vi "Loop_SM.vi"() -> ()   [LabVIEW 2017, in "WCDrive2018.lvlib"]
uses:
  WCDrive2018.lvlib
  ProtoType Code/EXAMPLE 2017 competition code/roboRIO Code/TypeDefs/Cluster_PID Constants Standard.ctl
  Cluster_Auto Shut Off Ranges.ctl
  ENUM_State.ctl
  Enum_SM Cmd Select.ctl
  ENUM_Action.ctl
  Enum Tab_Select PID Mode.ctl
  Cluster_SM to HW Data.ctl
  Enum_HW Cmd Select.ctl
  Cluster_CMD to SM Data.ctl
  Cluster_HW Status.ctl
  ProtoType Code/EXAMPLE 2017 competition code/roboRIO Code/TypeDefs/Cluster_SRX Status With Encoder.ctl
  Cluster_SM Status.ctl
  <vilib>/Rock Robotics/WPI/ThirdParty/Sensors/navX/_TypeDefs/FRIC_navX_DeviceNumbersTypeDef.ctl
  Global_CMD to SM Data.vi
  Global_HW_Status Out.vi
  _SHARE ALL/Global Share All/Global_STOP.vi
  <vilib>/addons/control/pid/pid.llb/PID (DBL).vi
  Global_SM Out Data.vi
  <vilib>/addons/control/pid/NI_PID_pid.lvlib
panel:
  out "Drive_HW_Status":T1
  out "SM Cmd":T3
  out "HW Cmd Out":T5
  in  "PID Select":T7
  in  "PID Track Rotation":T8={"proportional gain (Kc)"=0.005, "integral time (Ti, min)"=0.0, "derivative time (Td, min)"=0.0028} {"derivative time (Td, min)" format="%.5f"; "integral time (Ti, min)" format="%.5f"; "proportional gain (Kc)" format="%.5f"}
  in  "PID Lock Angle Rotation":T8={"proportional gain (Kc)"=0.012, "integral time (Ti, min)"=0.0, "derivative time (Td, min)"=0.002} {"derivative time (Td, min)" format="%.5f"; "integral time (Ti, min)" format="%.5f"; "proportional gain (Kc)" format="%.5f"}
  in  "PID Track Distance":T8={"proportional gain (Kc)"=0.005, "integral time (Ti, min)"=0.0, "derivative time (Td, min)"=0.0} {"derivative time (Td, min)" format="%.5f"; "integral time (Ti, min)" format="%.5f"; "proportional gain (Kc)" format="%.5f"}
  out "Action":T9
  out "CMDMODE":T4
  out "Complete":bool
  out "PID Output":dbl
  out "PID Reading":dbl
  out "PID Target":dbl
  out "Cycle Time":dbl
  out "State":T10
  out "Output":dbl(graph)
  out "Process Chart":cluster{"PID Target":dbl, "PID Reading":dbl}(graph)
  in  "Auto Shut Off Ranges":T11={"Track Front Back"=1.0, "Track Rotation"=1.0, "Track Lateral"=1.0, "Track Vision"=2.0}
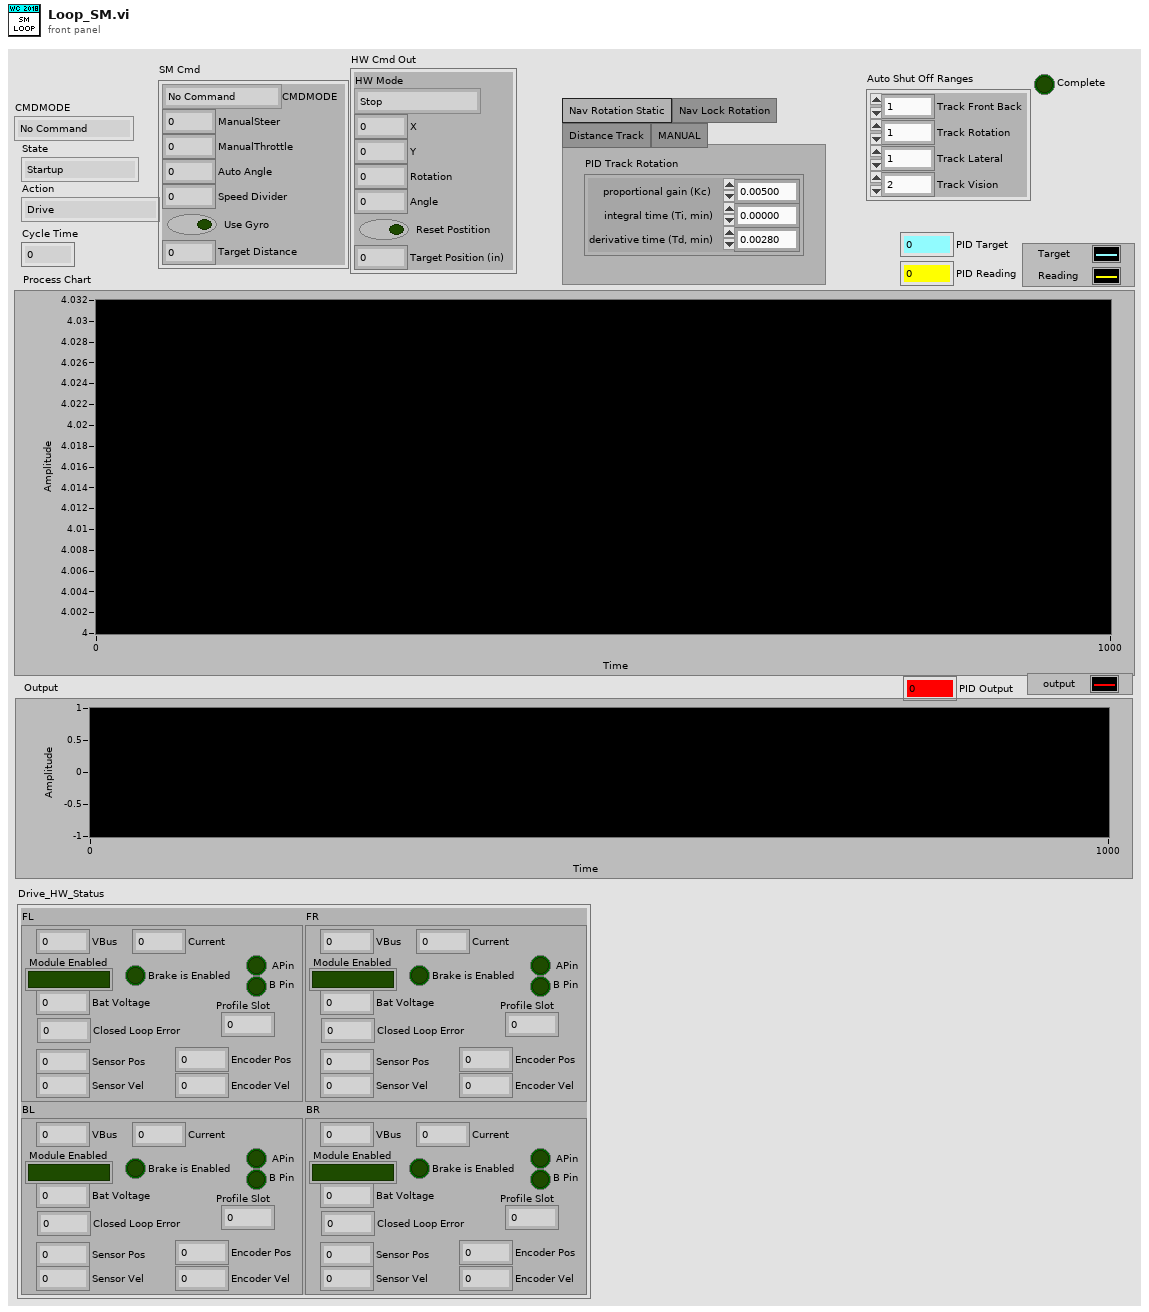
[diagram p1: front panel]
types:
  T1 = typedef "WCDrive2018.lvlib/Cluster_HW Status.ctl" = cluster{"BL":T2, "BR":T2, "FL":T2, "FR":T2}
  T2 = typedef "Cluster_SRX Status With Encoder.ctl" = cluster{"VBus ":dbl, "Module Enabled":bool, "Closed Loop Error":dbl, "Sensor Pos":dbl, "Sensor Vel":dbl, "Current":dbl, "Brake is Enabled":bool, "Encoder Pos":dbl, "Encoder Vel":dbl, " APin":bool, "B Pin":bool, "Bat Voltage":dbl, "Profile Slot":dbl}
  T3 = typedef "WCDrive2018.lvlib/Cluster_CMD to SM Data.ctl" = cluster{"CMDMODE":T4, "ManualSteer":dbl, "ManualThrottle":dbl, "Auto Angle":dbl, "Speed Divider":dbl, "Use Gyro":bool, "Target Distance":dbl}
  T4 = typedef "WCDrive2018.lvlib/Enum_SM Cmd Select.ctl" = enum16{"No Command", "Halt", "Manual Keep Rotation", "Manual", "Track Front", "Track Rotation"}
  T5 = typedef "WCDrive2018.lvlib/Cluster_SM to HW Data.ctl" = cluster{"HW Mode":T6, "X":dbl, "Y":dbl, "Rotation":dbl, "Angle":dbl, "Reset Postition":bool, "Target Position (in)":dbl}
  T6 = typedef "WCDrive2018.lvlib/Enum_HW Cmd Select.ctl" = enum16{"Stop", "Vbus", "Positon Lateral", "Postition  FrontBack"}
  T7 = typedef "WCDrive2018.lvlib/Enum Tab_Select PID Mode.ctl" = enum32{"Nav Rotation Static", "Nav Lock Rotation", "Distance Track", "MANUAL"}
  T8 = typedef "Cluster_PID Constants Standard.ctl" = cluster{"proportional gain (Kc)":dbl, "integral time (Ti, min)":dbl, "derivative time (Td, min)":dbl}
  T9 = typedef "WCDrive2018.lvlib/ENUM_Action.ctl" = enum16{"Drive", "No Action", "Manuel Keep Rotation", "Reset Time", "Stop Move", "Track Front Distance", "Set Lock Angle", "Reset Gyro", "Track Rotation", "NavX Pos Reset", "Reset Position"}
  T10 = typedef "WCDrive2018.lvlib/ENUM_State.ctl" = enum16{"Startup", "Idle", "Manual", "Rotation Tracking", "Distance Tracking", "Shutdown", "Manual Keep Rotation", "Halt"}
  T11 = typedef "WCDrive2018.lvlib/Cluster_Auto Shut Off Ranges.ctl" = cluster{"Track Front Back":dbl, "Track Rotation":dbl, "Track Lateral":dbl, "Track Vision":dbl}
  T12 = typedef "WCDrive2018.lvlib/Cluster_SM Status.ctl" = cluster{"Drive Cmd":T4, "Complete":bool}
  T13 = cluster{"Velocity X":dbl, "Velocity Y":dbl, "Velocity Z":dbl, "Displacement X":dbl, "Displacement Y":dbl, "Displacement Z":dbl}
  T14 = cluster{"Actions":T9[], "State":T10, "Current Time":timestamp, "Start Time":timestamp, "Loop Time (ms)":u32, "CMD Drive":T3, "Set Angle Out":dbl, "Sonar Distance":dbl, "Lock Angle":dbl, "previous State":T10, "Position Data":cluster{"Velocity X":dbl, "Velocity Y":dbl, "Velocity Z":dbl, "Displacement X":dbl, "Displacement Y":dbl, "Displacement Z":dbl}, "Shut Off Ranges":T11, "Status OUT":T12, "PID Target":dbl, "PID Reading":dbl, "PID Output":dbl, "DriveHWCmd":T5, "Gyro Angle":dbl, "Drive HW Status":T1, "PID Select":T7}
  T15 = typedef "FRIC_navX_DeviceNumbersTypeDef.ctl" = enum16{"Dev0", "Dev1", "Dev2", "Dev3"}
  T16 = cluster{"Yaw":dbl, "Roll":dbl, "Pitch":dbl, "Heading":dbl, "Fused Heading":dbl}
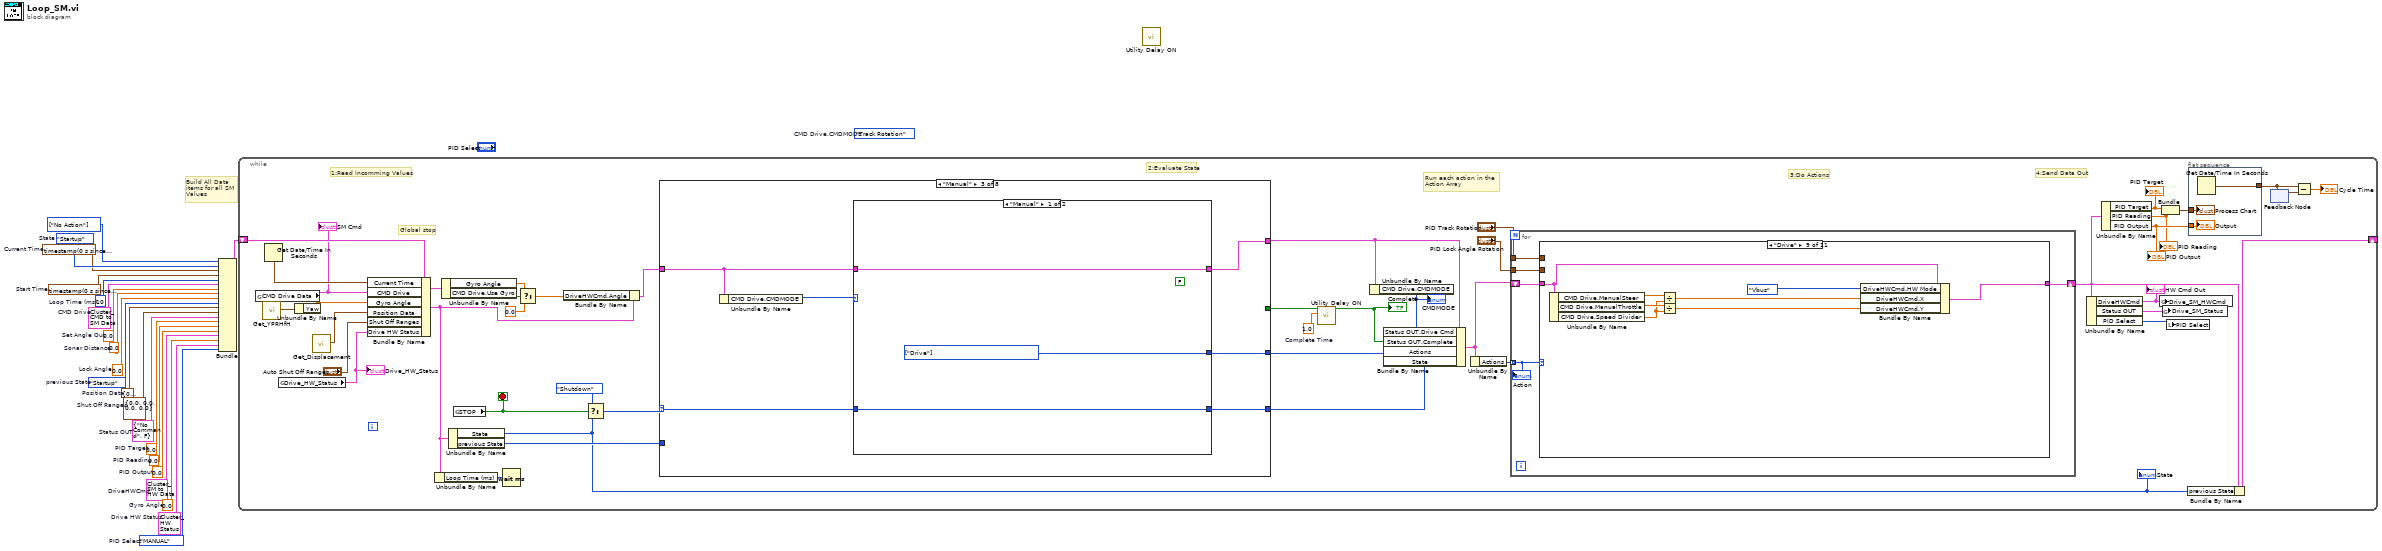
[diagram p0: block diagram]
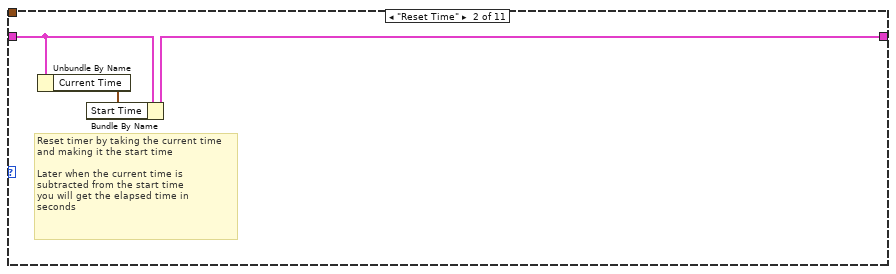
[diagram p3: hidden frame]
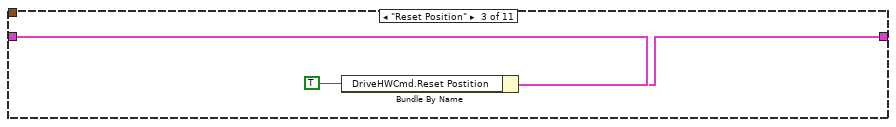
[diagram p4: hidden frame]
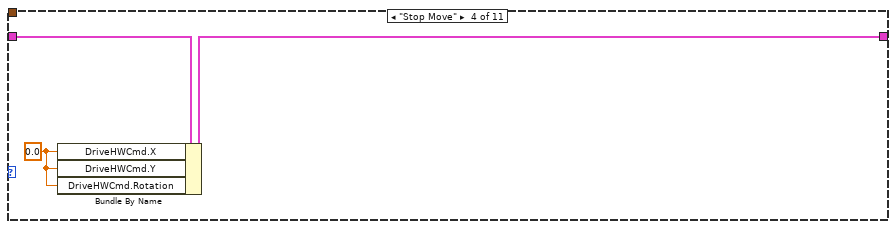
[diagram p5: hidden frame]
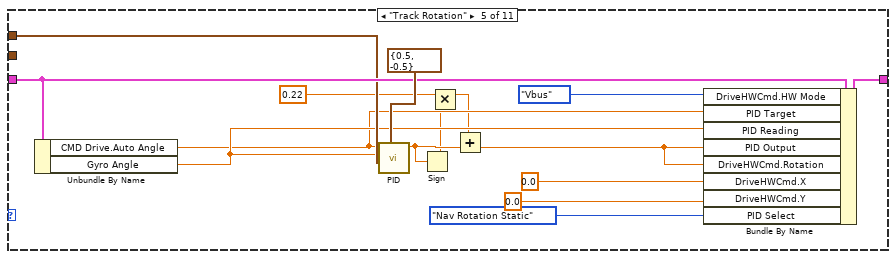
[diagram p6: hidden frame]
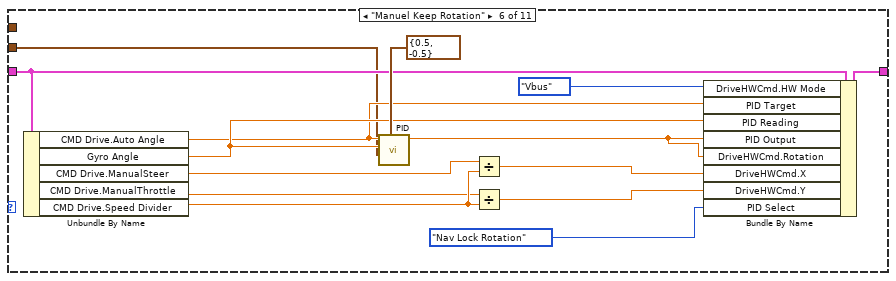
[diagram p7: hidden frame]
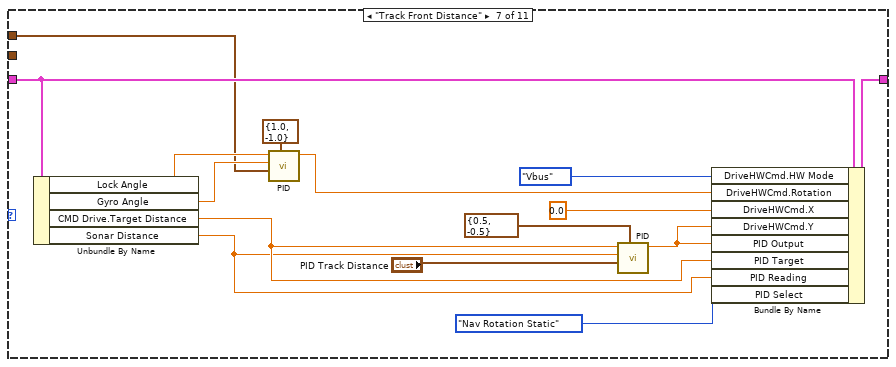
[diagram p8: hidden frame]
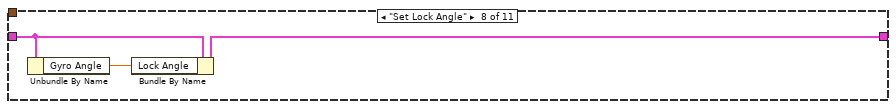
[diagram p9: hidden frame]
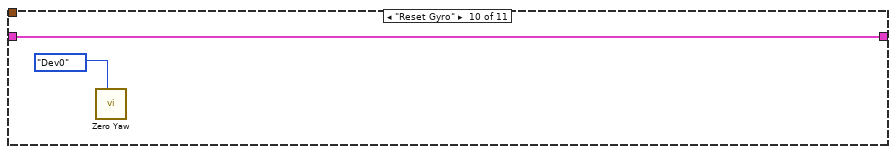
[diagram p10: hidden frame]
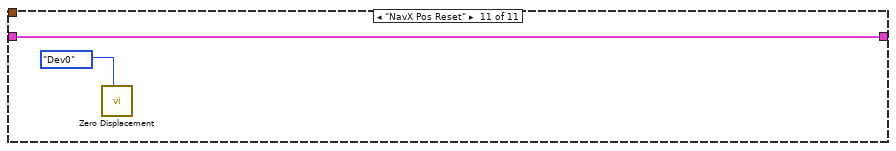
[diagram p11: hidden frame]
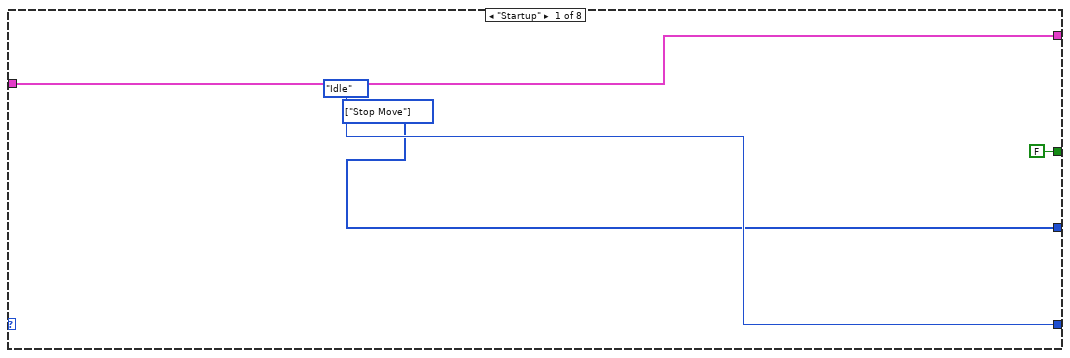
[diagram p12: hidden frame]
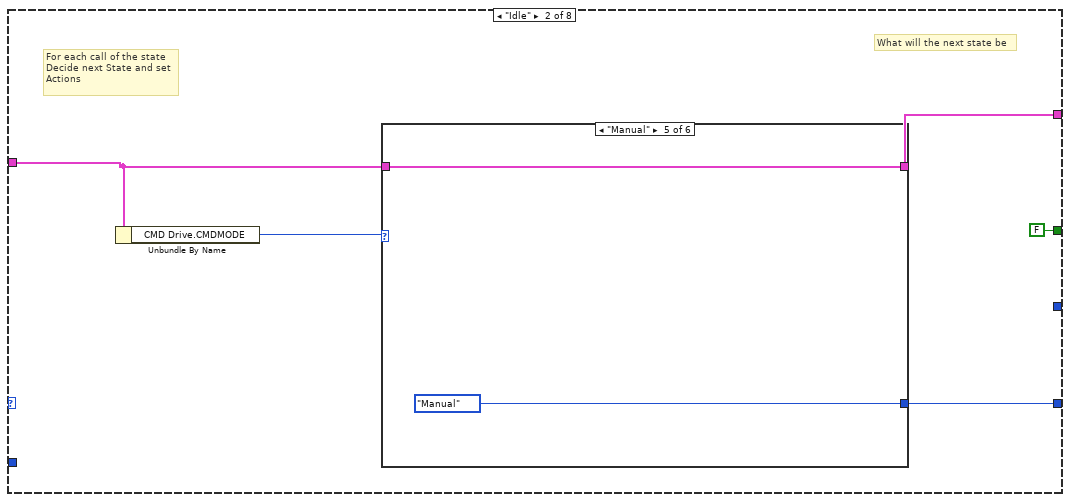
[diagram p13: hidden frame]
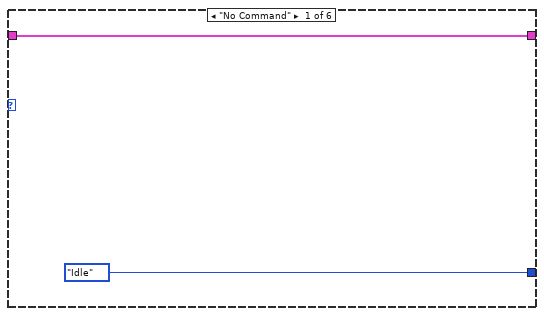
[diagram p14: hidden frame]
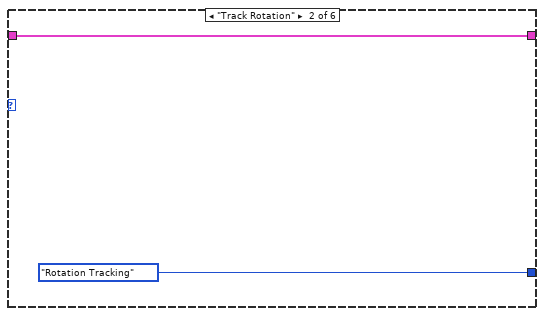
[diagram p15: hidden frame]
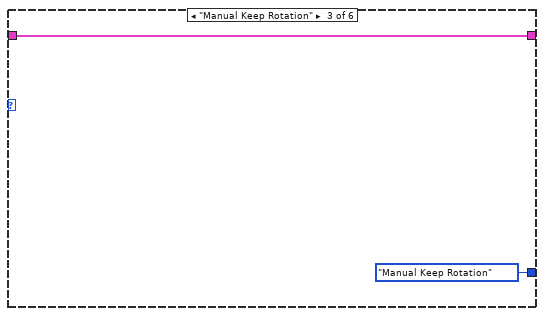
[diagram p16: hidden frame]
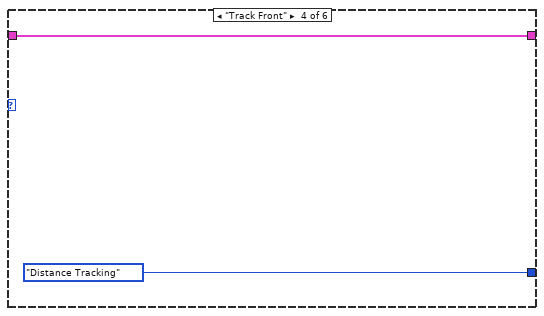
[diagram p17: hidden frame]
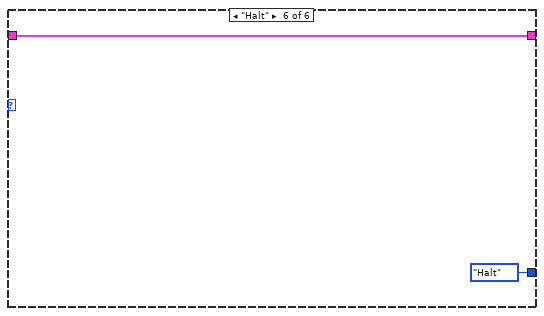
[diagram p18: hidden frame]
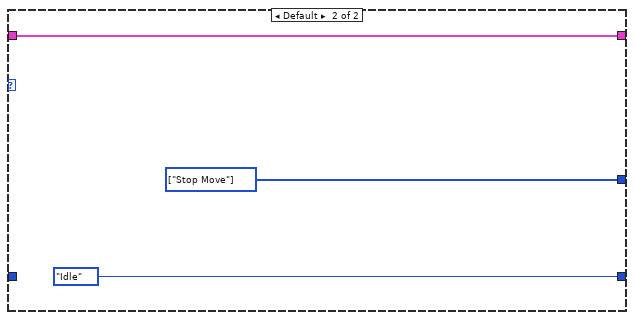
[diagram p19: hidden frame]
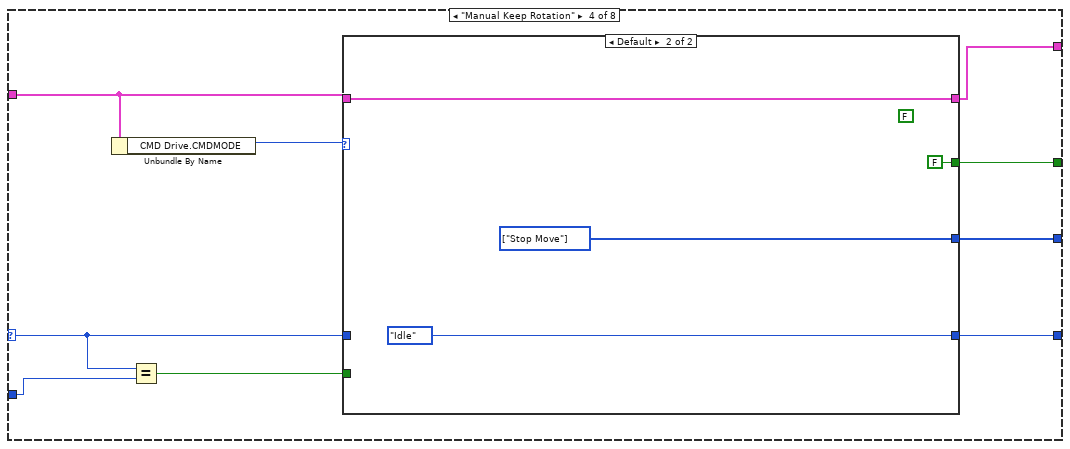
[diagram p20: hidden frame]
diagram:
  (unwired) Enum_SM_Cmd_Select."Track Rotation"  # CMD Drive.CMDMODE
  w1 = 0.0  # Sonar Distance
  w2 = Enum_Tab_Select_PID_Mode."MANUAL"  # PID Select
  w3 = T1 {"BL"={"VBus "=0.0, "Module Enabled"=FALSE, "Closed Loop Error"=0.0, "Sensor Pos"=0.0, "Sensor Vel"=0.0, "Current"=0.0, "Brake is Enabled"=FALSE, "Encoder Pos"=0.0, "Encoder Vel"=0.0, " APin"=FALSE, "B Pin"=FALSE, "Bat Voltage"=0.0, "Profile Slot"=0.0}, "BR"={"VBus "=0.0, "Module Enabled"=FALSE, "Closed Loop Error"=0.0, "Sensor Pos"=0.0, "Sensor Vel"=0.0, "Current"=0.0, "Brake is Enabled"=FALSE, "Encoder Pos"=0.0, "Encoder Vel"=0.0, " APin"=FALSE, "B Pin"=FALSE, "Bat Voltage"=0.0, "Profile Slot"=0.0}, "FL"={"VBus "=0.0, "Module Enabled"=FALSE, "Closed Loop Error"=0.0, "Sensor Pos"=0.0, "Sensor Vel"=0.0, "Current"=0.0, "Brake is Enabled"=FALSE, "Encoder Pos"=0.0, "Encoder Vel"=0.0, " APin"=FALSE, "B Pin"=FALSE, "Bat Voltage"=0.0, "Profile Slot"=0.0}, "FR"={"VBus "=0.0, "Module Enabled"=FALSE, "Closed Loop Error"=0.0, "Sensor Pos"=0.0, "Sensor Vel"=0.0, "Current"=0.0, "Brake is Enabled"=FALSE, "Encoder Pos"=0.0, "Encoder Vel"=0.0, " APin"=FALSE, "B Pin"=FALSE, "Bat Voltage"=0.0, "Profile Slot"=0.0}}  # Drive HW Status
  w4 = 0.0  # Gyro Angle
  w5 = T5 {"HW Mode"=enum."Postition  FrontBack", "X"=0.0, "Y"=0.0, "Rotation"=0.0, "Angle"=0.0, "Reset Postition"=FALSE, "Target Position (in)"=0.0}  # DriveHWCmd
  w6 = 0.0  # PID Output
  w7 = 0.0  # PID Reading
  w8 = 0.0  # PID Target
  w9 = T12 {"Drive Cmd"=enum."No Command", "Complete"=FALSE}  # Status OUT
  w10 = T11 {"Track Front Back"=0.0, "Track Rotation"=0.0, "Track Lateral"=0.0, "Track Vision"=0.0}  # Shut Off Ranges
  w11 = T13 {"Velocity X"=0.0, "Velocity Y"=0.0, "Velocity Z"=0.0, "Displacement X"=0.0, "Displacement Y"=0.0, "Displacement Z"=0.0}  # Position Data
  w12 = ENUM_State."Startup"  # previous State
  w13 = 0.0  # Lock Angle
  w14 = 0.0  # Set Angle Out
  w15 = T3 {"CMDMODE"=enum."No Command", "ManualSteer"=0.0, "ManualThrottle"=0.0, "Auto Angle"=0.0, "Speed Divider"=0.0, "Use Gyro"=FALSE, "Target Distance"=0.0}  # CMD Drive
  w16 = u32 10  # Loop Time (ms)
  w17 = T9[] [enum."No Action"] items=["Drive", "No Action", "Manuel Keep Rotation", "Reset Time", "Stop Move", "Track Front Distance", "Set Lock Angle", "Reset Gyro", "Track Rotation", "NavX Pos Reset", "Reset Position"] ("Actions")
  w18 = timestamp(0 s since 1904-01-01)  # Start Time
  w19 = timestamp(0 s since 1904-01-01)  # Current Time
  w20 = ENUM_State."Startup"  # State
  # "Build All Data items for all SM Values"
  n1 = Bundle("Actions"=w17, "State"=w20, "Current Time"=w19, "Start Time"=w18, "Loop Time (ms)"=w16, "CMD Drive"=w15, "Set Angle Out"=w14, "Sonar Distance"=w1, "Lock Angle"=w13, "previous State"=w12, "Position Data"=w11, "Shut Off Ranges"=w10, "Status OUT"=w9, "PID Target"=w8, "PID Reading"=w7, "PID Output"=w6, "DriveHWCmd"=w5, "Gyro Angle"=w4, "Drive HW Status"=w3, "PID Select"=w2) -> (w21:T14)  [unwired: 1 in]
  n2 = while {
    shift-right: [w45] -> _
    shift-left: w21 -> [w63]
    stop <- w61 stop-if-true
    w24 = 1.0  # Complete Time
    # "Run each action in the Action Array"
    # "1:Read Incomming Values"
    # "2:Evaluate State"
    # "3:Do Actions"
    # "4:Send Data Out"
    # "Global stop"
    n3 = global read "Global_CMD to SM Data.vi" "CMD Drive Data"() -> (w57:T3)
    "SM Cmd" <- w57
    n4 = call <vilib>:"Get_YPRHfH.vi"() -> ("YRPHfH"=w56:T16)  [unwired: 11 in]
    n5 = Get Date/Time In Seconds() -> (seconds since 1Jan1904=w62:timestamp)
    n6 = global read "Global_HW_Status Out.vi" "Drive_HW_Status"() -> (w27:T1)
    "Drive_HW_Status" <- w27
    n7 = Unbundle By Name(w56) -> ("Yaw"=w54:dbl)
    n8 = call <vilib>:"Get_Displacement.vi"() -> ("Displacement"=w44:T13)  [unwired: 11 in]
    n9 = Bundle By Name(cluster=w63, "Current Time"=w62, "CMD Drive"=w57, "Gyro Angle"=w54, "Position Data"=w44, "Shut Off Ranges"="Auto Shut Off Ranges", "Drive HW Status"=w27) -> (w49:T14)
    n10 = Unbundle By Name(w49) -> ("Loop Time (ms)"=w58:u32)
    n11 = Unbundle By Name(w49) -> ("Gyro Angle"=w51:dbl, "CMD Drive.Use Gyro"=w52:bool)
    n12 = Unbundle By Name(w49) -> ("State"=w43:T10, "previous State"=w46:T10)
    "State" <- w43
    n13 = global read "Global_STOP.vi" "STOP"() -> (w61:bool)
    n14 = Wait (ms)(milliseconds to wait=w58) -> ()  [unwired: 1 out]
    n15 = Select(t=w51, s=w52, f=0.0) -> (s? t:f=w47:dbl)
    n16 = Bundle By Name(cluster=w49, "DriveHWCmd.Angle"=w47) -> (w48:T14)
    n17 = Select(t=ENUM_State."Shutdown" ("State"), s=w61, f=w43) -> (s? t:f=w59:T10)
    n18 = case shown="\"Manual\"" w59 {
      selector: w59 -> [_ _ w167 w178 w196 w219 _ _]
      tunnel: w48 -> [w145 w149 w163 w179 w200 w222 w242 w245]
      tunnel: [w145 w148 w164 w180 w199 w221 w242 w245] -> w40
      tunnel: [ENUM_State."Idle" ("State") w147 w166 w182 w198 w218 ENUM_State."Shutdown" ("State") w244] -> w38
      tunnel: [w143 _ w165 w181 w197 w220 w240 w247] -> w55
      tunnel: w46 -> [_ _ _ w177 _ _ _ _]
      tunnel: [FALSE FALSE _ w175 w195 w217 FALSE w243] -> w23
      frame "Startup" {
        w143 = T9[] [enum."Stop Move"] items=["Drive", "No Action", "Manuel Keep Rotation", "Reset Time", "Stop Move", "Track Front Distance", "Set Lock Angle", "Reset Gyro", "Track Rotation", "NavX Pos Reset", "Reset Position"] ("Actions")
      }
      frame "Idle" {
        # "For each call of the state\nDecide next State and set\nActions"
        # "What will the next state be"
        n19 = Unbundle By Name(w149) -> ("CMD Drive.CMDMODE"=w150:T4)
        n20 = case shown="\"Manual\"" w150 {
          tunnel: w149 -> [w151 w153 w156 w157 w160 w162]
          tunnel: [w151 w153 w156 w157 w160 w162] -> w148
          tunnel: [ENUM_State."Idle" ("State") ENUM_State."Rotation Tracking" ("State") ENUM_State."Manual Keep Rotation" ("State") ENUM_State."Distance Tracking" ("State") ENUM_State."Manual" ("State") ENUM_State."Halt" ("State")] -> w147
          frame "No Command" {
          }
          frame "Track Rotation" {
          }
          frame "Manual Keep Rotation" {
          }
          frame "Track Front" {
          }
          frame "Manual" {
          }
          frame "Halt" {
          }
        }
      }
      frame "Manual" {
        (unwired) FALSE
        n21 = Unbundle By Name(w163) -> ("CMD Drive.CMDMODE"=w168:T4)
        n22 = case shown="\"Manual\"" w168 {
          tunnel: w163 -> [w170 w174]
          tunnel: [w170 w174] -> w164
          tunnel: [w169 ENUM_State."Idle" ("State")] -> w166
          tunnel: [w171 w172] -> w165
          tunnel: w167 -> [w169 _]
          frame "Manual" {
            w171 = T9[] [enum."Drive"] items=["Drive", "No Action", "Manuel Keep Rotation", "Reset Time", "Stop Move", "Track Front Distance", "Set Lock Angle", "Reset Gyro", "Track Rotation", "NavX Pos Reset", "Reset Position"] ("Actions")
          }
          frame Default {
            w172 = T9[] [enum."Stop Move"] items=["Drive", "No Action", "Manuel Keep Rotation", "Reset Time", "Stop Move", "Track Front Distance", "Set Lock Angle", "Reset Gyro", "Track Rotation", "NavX Pos Reset", "Reset Position"] ("Actions")
          }
        }
      }
      frame "Manual Keep Rotation" {
        (unwired) FALSE
        n23 = Unbundle By Name(w179) -> ("CMD Drive.CMDMODE"=w183:T4)
        n24 = Equal?(x=w178, y=w177) -> (x = y?=w176:bool)
        n25 = case shown="Default" w183 {
          tunnel: w179 -> [w187 w194]
          tunnel: [w187 w194] -> w180
          tunnel: [w186 ENUM_State."Idle" ("State")] -> w182
          tunnel: [w188 w192] -> w181
          tunnel: w178 -> [w186 _]
          tunnel: w176 -> [w185 _]
          tunnel: [FALSE FALSE] -> w175
          frame "Manual Keep Rotation" {
            n26 = case shown="False" w185 {
              tunnel: [w189 w190] -> w188
              frame True {
                w189 = T9[] [enum."Manuel Keep Rotation"] items=["Drive", "No Action", "Manuel Keep Rotation", "Reset Time", "Stop Move", "Track Front Distance", "Set Lock Angle", "Reset Gyro", "Track Rotation", "NavX Pos Reset", "Reset Position"] ("Actions")
              }
              frame False {
                w190 = T9[] [enum."Manuel Keep Rotation", enum."Set Lock Angle"] items=["Drive", "No Action", "Manuel Keep Rotation", "Reset Time", "Stop Move", "Track Front Distance", "Set Lock Angle", "Reset Gyro", "Track Rotation", "NavX Pos Reset", "Reset Position"] ("Actions")
              }
            }
          }
          frame Default {
            w192 = T9[] [enum."Stop Move"] items=["Drive", "No Action", "Manuel Keep Rotation", "Reset Time", "Stop Move", "Track Front Distance", "Set Lock Angle", "Reset Gyro", "Track Rotation", "NavX Pos Reset", "Reset Position"] ("Actions")
          }
        }
      }
      frame "Rotation Tracking" {
        n27 = Unbundle By Name(w200) -> ("CMD Drive.CMDMODE"=w201:T4)
        n28 = case shown="Default" w201 {
          tunnel: w200 -> [w203 w216]
          tunnel: [w203 w216] -> w199
          tunnel: [w205 ENUM_State."Idle" ("State")] -> w198
          tunnel: [w204 w214] -> w197
          tunnel: [w202 FALSE] -> w195
          tunnel: w196 -> [w205 _]
          frame "Track Rotation" {
            n29 = Unbundle By Name(w203) -> ("CMD Drive.Auto Angle"=w209:dbl, "Gyro Angle"=w210:dbl, "Shut Off Ranges.Track Rotation"=w207:dbl)
            n30 = Subtract(x=w209, y=w210) -> (x-y=w208:dbl)
            n31 = Absolute Value(x=w208) -> (abs(x)=w206:dbl)
            n32 = Less Or Equal?(x=w206, y=w207) -> (x <= y?=w202:bool)
            n33 = case shown="True" w202 {
              tunnel: [w211 w212] -> w204
              frame False {
                w211 = T9[] [enum."Track Rotation"] items=["Drive", "No Action", "Manuel Keep Rotation", "Reset Time", "Stop Move", "Track Front Distance", "Set Lock Angle", "Reset Gyro", "Track Rotation", "NavX Pos Reset", "Reset Position"] ("Actions")
              }
              frame True {
                w212 = T9[] [enum."Stop Move"] items=["Drive", "No Action", "Manuel Keep Rotation", "Reset Time", "Stop Move", "Track Front Distance", "Set Lock Angle", "Reset Gyro", "Track Rotation", "NavX Pos Reset", "Reset Position"] ("Actions")
              }
            }
          }
          frame Default {
            w214 = T9[] [enum."Stop Move"] items=["Drive", "No Action", "Manuel Keep Rotation", "Reset Time", "Stop Move", "Track Front Distance", "Set Lock Angle", "Reset Gyro", "Track Rotation", "NavX Pos Reset", "Reset Position"] ("Actions")
          }
        }
      }
      frame "Distance Tracking" {
        n34 = Unbundle By Name(w222) -> ("CMD Drive.CMDMODE"=w223:T4)
        n35 = case shown="Default" w223 {
          tunnel: w222 -> [w231 w238]
          tunnel: [w231 w238] -> w221
          tunnel: [w226 ENUM_State."Idle" ("State")] -> w218
          tunnel: [w232 w236] -> w220
          tunnel: [w228 FALSE] -> w217
          tunnel: w219 -> [w226 _]
          frame "Track Front" {
            n36 = Unbundle By Name(w231) -> ("CMD Drive.Target Distance"=w230:dbl, "Sonar Distance"=w225:dbl, "Shut Off Ranges.Track Rotation"=w224:dbl)
            n37 = Subtract(x=w230, y=w225) -> (x-y=w229:dbl)
            n38 = Absolute Value(x=w229) -> (abs(x)=w227:dbl)
            n39 = Less Or Equal?(x=w227, y=w224) -> (x <= y?=w228:bool)
            n40 = case shown="False" w228 {
              tunnel: [w233 w234] -> w232
              frame False {
                w233 = T9[] [enum."Track Front Distance"] items=["Drive", "No Action", "Manuel Keep Rotation", "Reset Time", "Stop Move", "Track Front Distance", "Set Lock Angle", "Reset Gyro", "Track Rotation", "NavX Pos Reset", "Reset Position"] ("Actions")
              }
              frame True {
                w234 = T9[] [enum."Stop Move"] items=["Drive", "No Action", "Manuel Keep Rotation", "Reset Time", "Stop Move", "Track Front Distance", "Set Lock Angle", "Reset Gyro", "Track Rotation", "NavX Pos Reset", "Reset Position"] ("Actions")
              }
            }
          }
          frame Default {
            w236 = T9[] [enum."Stop Move"] items=["Drive", "No Action", "Manuel Keep Rotation", "Reset Time", "Stop Move", "Track Front Distance", "Set Lock Angle", "Reset Gyro", "Track Rotation", "NavX Pos Reset", "Reset Position"] ("Actions")
          }
        }
      }
      frame "Shutdown" {
        w240 = T9[] [enum."Stop Move"] items=["Drive", "No Action", "Manuel Keep Rotation", "Reset Time", "Stop Move", "Track Front Distance", "Set Lock Angle", "Reset Gyro", "Track Rotation", "NavX Pos Reset", "Reset Position"] ("Actions")
      }
      frame "Halt" {
        (unwired) FALSE
        n41 = Unbundle By Name(w245) -> ("CMD Drive.CMDMODE"=w246:T4)
        n42 = case shown="\"Halt\"" w246 {
          tunnel: [ENUM_State."Halt" ("State") ENUM_State."Idle" ("State")] -> w244
          tunnel: [w250 w252] -> w247
          tunnel: [FALSE FALSE] -> w243
          frame "Halt" {
            w250 = T9[] [enum."Stop Move"] items=["Drive", "No Action", "Manuel Keep Rotation", "Reset Time", "Stop Move", "Track Front Distance", "Set Lock Angle", "Reset Gyro", "Track Rotation", "NavX Pos Reset", "Reset Position"] ("Actions")
          }
          frame Default {
            w252 = T9[] [enum."Stop Move"] items=["Drive", "No Action", "Manuel Keep Rotation", "Reset Time", "Stop Move", "Track Front Distance", "Set Lock Angle", "Reset Gyro", "Track Rotation", "NavX Pos Reset", "Reset Position"] ("Actions")
          }
        }
      }
    }
    n43 = call "Utility Delay ON.vi"("Delay Time"=w24, "Input"=w23) -> ("Output"=w25:bool)  [unwired: 9 in]
    "Complete" <- w25
    n44 = Unbundle By Name(w40) -> ("CMD Drive.CMDMODE"=w39:T4)
    "CMDMODE" <- w39
    n45 = Bundle By Name(cluster=w40, "Status OUT.Drive Cmd"=w39, "Status OUT.Complete"=w25, "Actions"=w55, "State"=w38) -> (w22:T14)
    n46 = Unbundle By Name(w22) -> ("Actions"=w64:T9[])
    n47 = for {
      tunnel: w64 -> [w72] mode=indexing
      shift-right: [w71] -> w36
      shift-left: w22 -> [w70]
      tunnel: "PID Track Rotation" -> [w69]
      tunnel: "PID Lock Angle Rotation" -> [w68]
      n48 = case shown="\"Drive\"" w72 {
        tunnel: w70 -> [w73 w76 w79 w82 w95 w109 w124 w129 w137 w139 w141]
        tunnel: [w73 w75 w78 w81 w96 w110 w125 w128 w136 w139 w141] -> w71
        tunnel: w69 -> [_ _ _ _ w93 _ w117 _ _ _ _]
        tunnel: w68 -> [_ _ _ _ _ w99 _ _ _ _ _]
        frame "No Action" {
        }
        frame "Reset Time" {
          # "Reset timer by taking the current time\nand making it the start time\n\nLater when the current time is \nsubtracted from the start time\nyou will get the elapsed time in \nseconds"
          n49 = Unbundle By Name(w76) -> ("Current Time"=w74:timestamp)
          n50 = Bundle By Name(cluster=w76, "Start Time"=w74) -> (w75:T14)
        }
        frame "Reset Position" {
          n51 = Bundle By Name(cluster=w79, "DriveHWCmd.Reset Postition"=TRUE ("DriveHWCmd OUT.Reset Postition")) -> (w78:T14)
        }
        frame "Stop Move" {
          w80 = 0.0 ("Drive Data.X")
          n52 = Bundle By Name(cluster=w82, "DriveHWCmd.X"=w80, "DriveHWCmd.Y"=w80, "DriveHWCmd.Rotation"=w80) -> (w81:T14)
        }
        frame "Track Rotation" {
          n53 = Unbundle By Name(w95) -> ("CMD Drive.Auto Angle"=w91:dbl, "Gyro Angle"=w92:dbl)
          n54 = call-poly <vilib>:"PID.vi"("output range"=cluster{"output high":dbl, "output low":dbl} {"output high"=0.5, "output low"=-0.5} ("ROITATION range"), "PID gains"=w93, "process variable"=w92, "setpoint"=w91) -> ("output"=w86:dbl)  [unwired: 6 in, 1 out]
          n55 = Sign(1:w86) -> (0:w85:dbl)
          n56 = Multiply(x=0.22, y=w85) -> (x*y=w87:dbl)
          n57 = Add(x=w87, y=w86) -> (x+y=w89:dbl)
          n58 = Bundle By Name(cluster=w95, "DriveHWCmd.HW Mode"=Enum_HW_Cmd_Select."Vbus" ("HWCMD Out.HW Mode"), "PID Target"=w91, "PID Reading"=w92, "PID Output"=w89, "DriveHWCmd.Rotation"=w89, "DriveHWCmd.X"=0.0 ("HWCMD Out.X"), "DriveHWCmd.Y"=0.0 ("HWCMD Out.X"), "PID Select"=Enum_Tab_Select_PID_Mode."Nav Rotation Static") -> (w96:T14)
        }
        frame "Manuel Keep Rotation" {
          n59 = Unbundle By Name(w109) -> ("CMD Drive.Auto Angle"=w102:dbl, "Gyro Angle"=w103:dbl, "CMD Drive.ManualSteer"=w104:dbl, "CMD Drive.ManualThrottle"=w105:dbl, "CMD Drive.Speed Divider"=w106:dbl)
          n60 = call-poly <vilib>:"PID.vi"("output range"=cluster{"output high":dbl, "output low":dbl} {"output high"=0.5, "output low"=-0.5} ("ROITATION range"), "PID gains"=w99, "process variable"=w103, "setpoint"=w102) -> ("output"=w100:dbl)  [unwired: 6 in, 1 out]
          n61 = Divide(x=w104, y=w106) -> (x/y=w107:dbl)
          n62 = Divide(x=w105, y=w106) -> (x/y=w108:dbl)
          n63 = Bundle By Name(cluster=w109, "DriveHWCmd.HW Mode"=Enum_HW_Cmd_Select."Vbus" ("HWCMD Out.HW Mode"), "PID Target"=w102, "PID Reading"=w103, "PID Output"=w100, "DriveHWCmd.Rotation"=w100, "DriveHWCmd.X"=w107, "DriveHWCmd.Y"=w108, "PID Select"=Enum_Tab_Select_PID_Mode."Nav Lock Rotation") -> (w110:T14)
        }
        frame "Track Front Distance" {
          n64 = Unbundle By Name(w124) -> ("Lock Angle"=w122:dbl, "Gyro Angle"=w123:dbl, "CMD Drive.Target Distance"=w114:dbl, "Sonar Distance"=w112:dbl)
          n65 = call-poly <vilib>:"PID.vi"("output range"=cluster{"output high":dbl, "output low":dbl} {"output high"=1.0, "output low"=-1.0}, "PID gains"=w117, "process variable"=w123, "setpoint"=w122) -> ("output"=w121:dbl)  [unwired: 6 in, 1 out]
          n66 = call-poly <vilib>:"PID.vi"("output range"=cluster{"output high":dbl, "output low":dbl} {"output high"=0.5, "output low"=-0.5}, "PID gains"="PID Track Distance", "process variable"=w112, "setpoint"=w114) -> ("output"=w116:dbl)  [unwired: 6 in, 1 out]
          n67 = Bundle By Name(cluster=w124, "DriveHWCmd.HW Mode"=Enum_HW_Cmd_Select."Vbus" ("HWCMD Out.HW Mode"), "DriveHWCmd.Rotation"=w121, "DriveHWCmd.X"=0.0 ("X Out"), "DriveHWCmd.Y"=w116, "PID Output"=w116, "PID Target"=w114, "PID Reading"=w112, "PID Select"=Enum_Tab_Select_PID_Mode."Nav Rotation Static") -> (w125:T14)
        }
        frame "Set Lock Angle" {
          n68 = Unbundle By Name(w129) -> ("Gyro Angle"=w127:dbl)
          n69 = Bundle By Name(cluster=w129, "Lock Angle"=w127) -> (w128:T14)
        }
        frame "Drive" {
          n70 = Unbundle By Name(w137) -> ("CMD Drive.ManualSteer"=w131:dbl, "CMD Drive.ManualThrottle"=w133:dbl, "CMD Drive.Speed Divider"=w132:dbl)
          n71 = Divide(x=w131, y=w132) -> (x/y=w135:dbl)
          n72 = Divide(x=w133, y=w132) -> (x/y=w134:dbl)
          n73 = Bundle By Name(cluster=w137, "DriveHWCmd.HW Mode"=Enum_HW_Cmd_Select."Vbus" ("HWCMD Out.HW Mode"), "DriveHWCmd.X"=w135, "DriveHWCmd.Y"=w134) -> (w136:T14)
        }
        frame "Reset Gyro" {
          n74 = call <vilib>:"Zero Yaw.vi"("Device Number"=FRIC_navX_DeviceNumbersTypeDef."Dev0") -> ()  [unwired: 11 in]
        }
        frame "NavX Pos Reset" {
          n75 = call <vilib>:"Zero Displacement.vi"("Device Number"=FRIC_navX_DeviceNumbersTypeDef."Dev0") -> ()  [unwired: 11 in]
        }
      }
      "Action" <- w72
    }
    n76 = Unbundle By Name(w36) -> ("DriveHWCmd"=w53:T5, "Status OUT"=w41:T12, "PID Select"=w26:T7)
    "HW Cmd Out" <- w53
    n77 = Unbundle By Name(w36) -> ("PID Target"=w34:dbl, "PID Reading"=w33:dbl, "PID Output"=w35:dbl)
    "PID Target" <- w34
    "PID Reading" <- w33
    "PID Output" <- w35
    n78 = global write "Global_SM Out Data.vi" "Drive_SM_HWCmd"(w53) -> ()
    n79 = Bundle("PID Target"=w34, "PID Reading"=w33) -> (w32:cluster{"PID Target":dbl, "PID Reading":dbl})  [unwired: 1 in]
    n80 = global write "Global_SM Out Data.vi" "Drive_SM_Status"(w41) -> ()
    n81 = local write "PID Select"(w26) -> ()
    n82 = Bundle By Name(cluster=w36, "previous State"=w43) -> (w45:T14)
    n83 = flat-sequence {
      tunnel: w35 -> [w67]
      tunnel: w32 -> [w66]
      tunnel: [w65] -> w30
      frame #0 {
        n84 = Get Date/Time In Seconds() -> (seconds since 1Jan1904=w65:timestamp)
        "Process Chart" <- w66
        "Output" <- w67
      }
    }
    n85 = feedback-in #1(w30) -> ()
    n86 = feedback #1() -> (w31:timestamp)  [unwired: 1 in]
    n87 = Subtract(x=w30, y=w31) -> (x-y=→"Cycle Time":dbl)
  }
  n88 = call "Utility Delay ON.vi"() -> ()  [unwired: 11 in, 1 out]
